vi "Arcade Drive Straight Immediate Implementation.vi"(9 "Drive PID Gains":T1={"proportional gain (Kc)"=1.0, "integral time (Ti, min)"=0.01, "derivative time (Td, min)"=0.0} {"derivative time (Td, min)" format="%.3f"; "integral time (Ti, min)" format="%.3f"; "proportional gain (Kc)" format="%.3f"}, 10 "Left Setpoint":dbl, 11 "Angle Setpoint":dbl format="%.2f") -> (3 "Numeric":dbl)   [LabVIEW 2019]
uses:
  <vilib>/addons/control/pid/pid.llb/PID (DBL).vi
  <vilib>/addons/control/pid/NI_PID_pid.lvlib
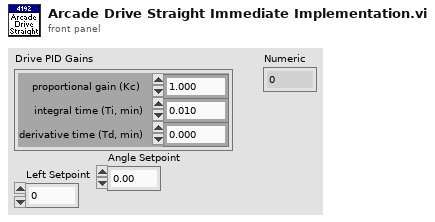
[diagram p1: front panel]
types:
  T1 = cluster{"proportional gain (Kc)":dbl, "integral time (Ti, min)":dbl, "derivative time (Td, min)":dbl}
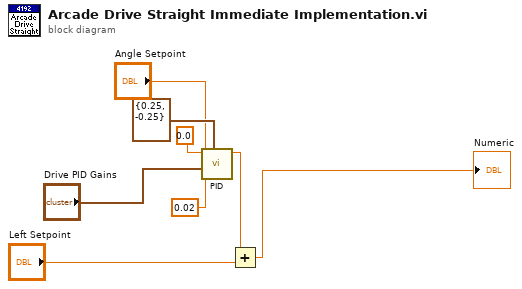
[diagram p0: block diagram]
diagram:
  n1 = call-poly <vilib>:"PID.vi"("output range"=cluster{"output high":dbl, "output low":dbl} {"output high"=0.25, "output low"=-0.25}, "dt (s)"=0.02, "PID gains"="Drive PID Gains", "process variable"="Angle Setpoint", "setpoint"=0.0 ("process variable")) -> ("output"=w5:dbl)  [unwired: 5 in, 1 out]
  n2 = Add(x=w5, y="Left Setpoint") -> (x+y=→"Numeric":dbl)
